vi "Main.vi"(11 "Module Admin":refnum<class "Delacor_lib_QMH_Cloneable Module Admin.lvclass">) -> ()   [LabVIEW 2019, in "moduloDqmh.lvlib"]
doc: "This template is based off of the Queued Message Handler design pattern and the Queued Message Handler project template that ships with LabVIEW.\n\nThe main difference is that the queue is private to this module and communication between modules is performed via Broadcast and Request events.\n\nRequest events are wrapped in public API methods and are handled in the Event Handling Loop (EHL) of this VI. Any module can register for Broadcast events sent by this module. The EHL generates messages based on user interface actions.\n\nThe Message Handling Loop (MHL) processes messages generated by the EHL, or by other messages. The messages are string values, so new messages can be added easily to the Message Cases case structure in the MHL. Each message cluster can also provide an optional value for Message Data, which is a variant that can be converted to whatever message-specific data is required.\n_____\nBased on Delacor QMH Project Template 5.0.0.82."
uses:
  moduloDqmh.lvlib
  <vilib>/Delacor/Delacor QMH/Libraries/Cloneable Module Admin_class/Delacor_lib_QMH_Cloneable Module Admin.lvclass
  C:/Program Files (x86)/National Instruments/LabVIEW 2019/vi.lib/Delacor/Delacor QMH/Libraries/Module Admin_class/Delacor_lib_QMH_Module Admin.lvclass
  Control 14.ctl
  Module Data--cluster.ctl
  <vilib>/Delacor/Delacor QMH/Libraries/Cloneable Module Admin_class/Delacor_lib_QMH_Cloneable Module Admin.lvclass/Delacor_lib_QMH_Cloneable Module Admin.ctl
  READ ADC Argument--cluster.ctl
  <vilib>/Delacor/Delacor QMH/Libraries/Message Queue_class/Delacor_lib_QMH_Message Queue.lvclass/Delacor_lib_QMH_Message Queue.ctl
  Read Port Argument--cluster.ctl
  Read Pin Argument--cluster.ctl
  Write Port Argument--cluster.ctl
  Write Pin Argument--cluster.ctl
  Stop Argument--cluster.ctl
  <vilib>/Delacor/Delacor QMH/Libraries/Module Admin_class/Delacor_lib_QMH_Module Admin.lvclass/Delacor_lib_QMH_Module Admin.ctl
  Arduino.lvclass
  E:/7to semestre/instrumentacion virtual/proyecto final/proyecto-final/Serial Device.lvclass
  NXP.lvclass
  simulado.lvclass
  <vilib>/Delacor/Delacor QMH/Libraries/Cloneable Module Admin_class/Delacor_lib_QMH_Get Module ID.vi
  <vilib>/Delacor/Delacor QMH/Libraries/Message Queue_class/Delacor_lib_QMH_Enqueue Message (Single).vi
  <vilib>/Delacor/Delacor QMH/Libraries/Module Admin_class/Delacor_lib_QMH_Get External Launch.vi
  <vilib>/Utility/error.llb/Error Cluster From Error Code.vi
  <vilib>/ErrorRing/Error Ring.xnode
  <vilib>/Delacor/Delacor QMH/Libraries/Message Queue_class/Delacor_lib_QMH_Message Queue.lvclass
  Serial Device.lvclass
panel:
  in  "VISA COM PORT":refnum<visa-resource-name>
  in  "Serial device Brand":T1
  in  "Config":bool
  out "Respuesta":string
  in  "CANAL":dbl
  in  "READ ADC":bool
  in  "VALOR":string
  in  "PORT":dbl
  in  "SET PORT":bool
  out "Array":bool[](array[boolean])
  in  "PORT 2":dbl
  in  "READ PORT":bool
  in  "Value":bool
  in  "PIN":dbl
  in  "PORT":dbl
  in  "SET PIN":bool
  out "Status":string
  out "Value PIN":bool
  in  "PIN":dbl
  in  "PORT":dbl
  in  "READ PIN":bool
  out "error out":errorcluster
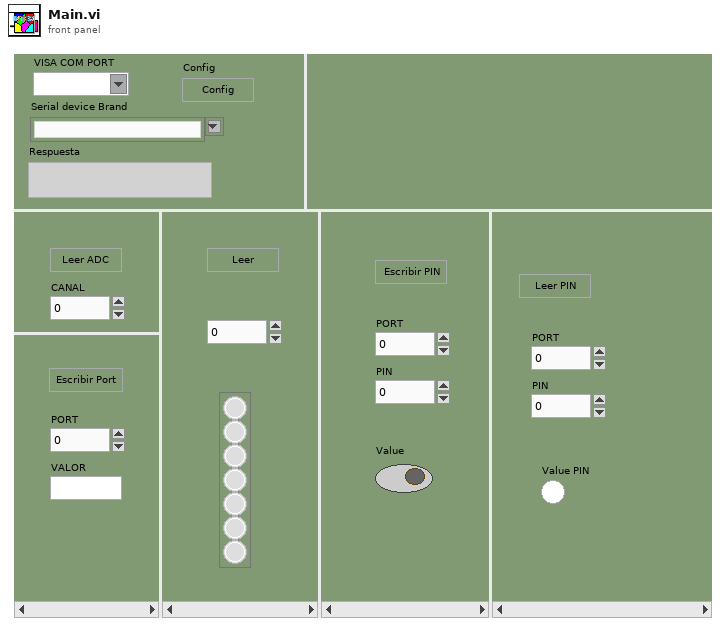
[diagram p1: front panel]
types:
  T1 = typedef "Serial Device.lvclass/Control 14.ctl" = string
  T2 = typedef "moduloDqmh.lvlib/Request Events--cluster.ctl" = cluster{"Stop Module":refnum<user-event>, "Show Panel":refnum<user-event>, "Hide Panel":refnum<user-event>, "Show Diagram":refnum<user-event>, "Get Module Execution Status":refnum<user-event>, "READ ADC":refnum<user-event>, "Read Port":refnum<user-event>, "Read Pin":refnum<user-event>, "Write Port":refnum<user-event>, "Write Pin":refnum<user-event>}
  T3 = typedef "moduloDqmh.lvlib/Module Data--cluster.ctl" = cluster{"Status":string}
  T4 = typedef "moduloDqmh.lvlib/READ ADC Argument--cluster.ctl" = cluster{"Module ID":i32, "CANAL":dbl}
  T5 = typedef "moduloDqmh.lvlib/Read Port Argument--cluster.ctl" = cluster{"Module ID":i32, "PORT 2":dbl}
  T6 = typedef "moduloDqmh.lvlib/Read Pin Argument--cluster.ctl" = cluster{"Module ID":i32, "PIN 2":dbl, "Port 4":dbl}
  T7 = typedef "moduloDqmh.lvlib/Write Port Argument--cluster.ctl" = cluster{"Module ID":i32, "String":string, "Numeric":dbl}
  T8 = typedef "moduloDqmh.lvlib/Write Pin Argument--cluster.ctl" = cluster{"Module ID":i32, "Port 3":dbl, "Pin":dbl, "Value":bool}
  T9 = enum32{"invalid lock state", "Not Locked", "Locked (No Password)", "Password-protected"}
  T10 = typedef "moduloDqmh.lvlib/Stop Argument--cluster.ctl" = cluster{"Module ID":i32, "Origin":string, "Exit via Stop Module Req?":bool, "Wait for Module to stop?":bool}
  T11 = enum32{"Invalid", "Standard", "Closed", "Hidden", "Minimized", "Maximized"}
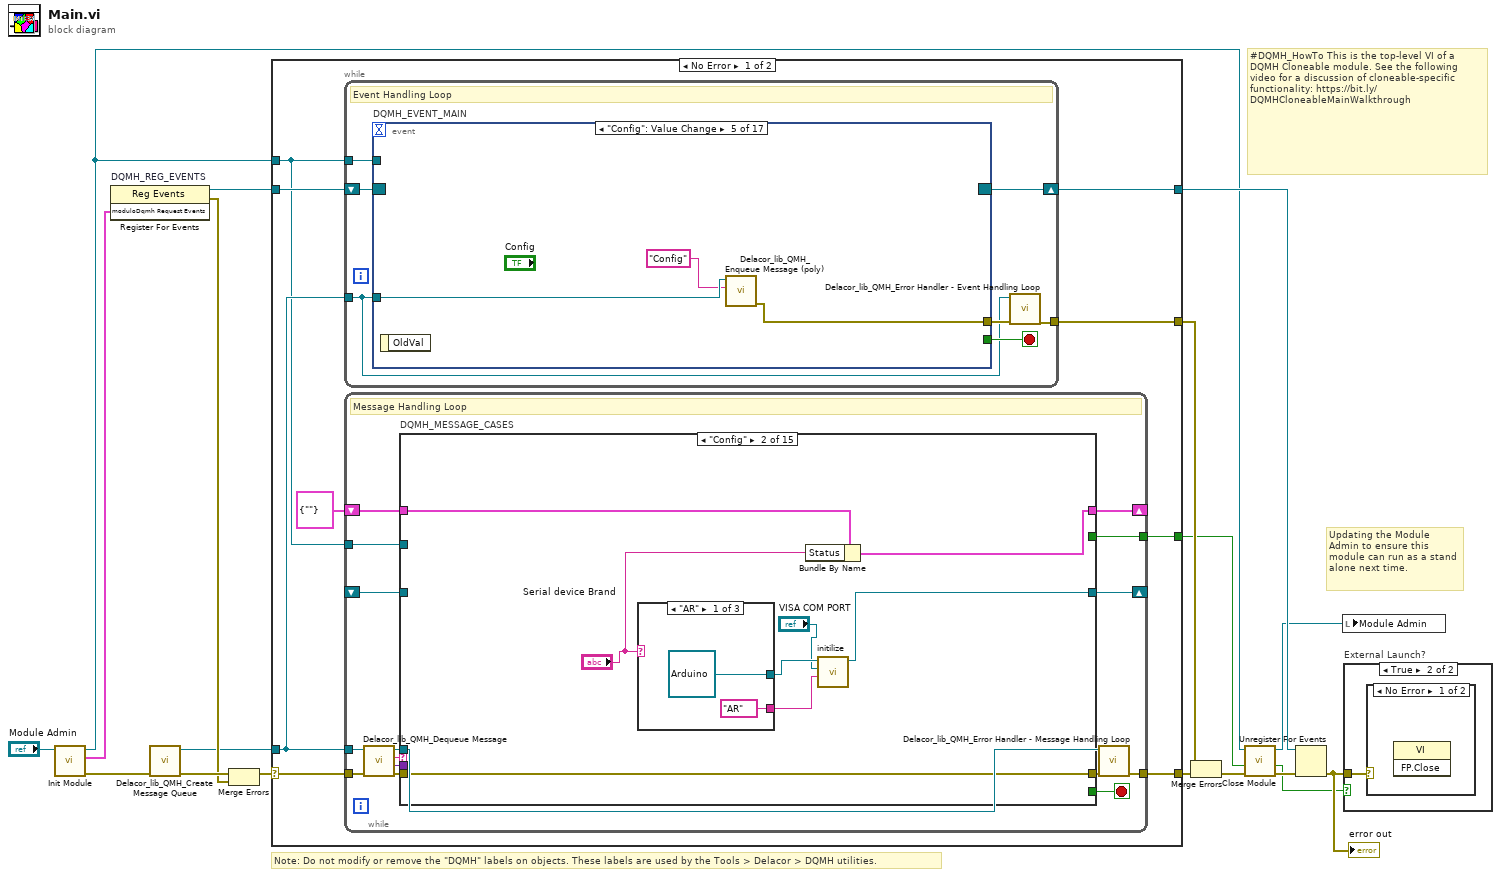
[diagram p0: block diagram]
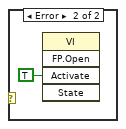
[diagram p3: hidden frame]
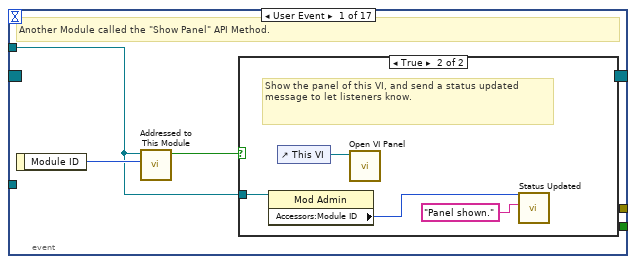
[diagram p4: hidden frame]
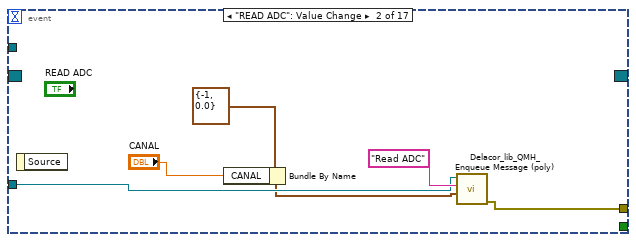
[diagram p6: hidden frame]
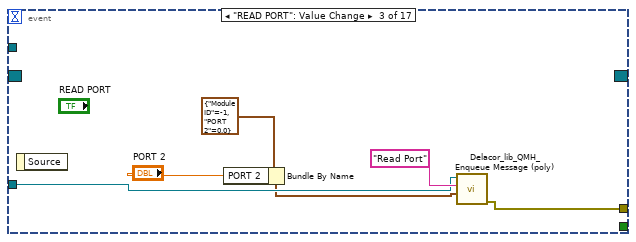
[diagram p7: hidden frame]
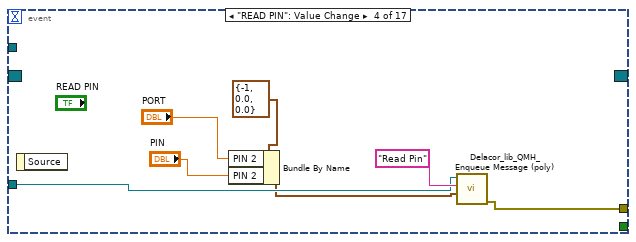
[diagram p8: hidden frame]
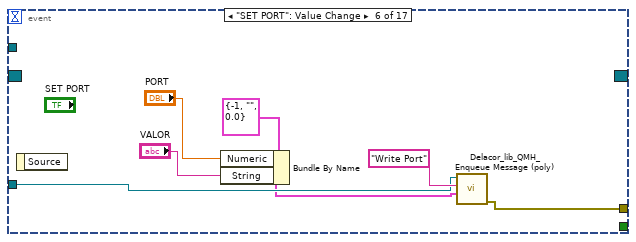
[diagram p9: hidden frame]
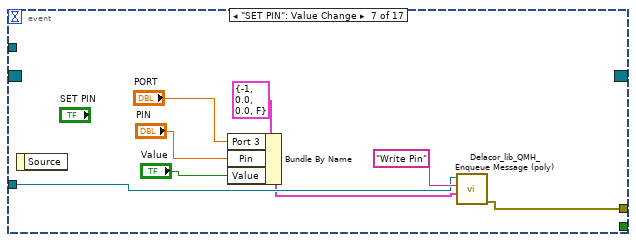
[diagram p10: hidden frame]
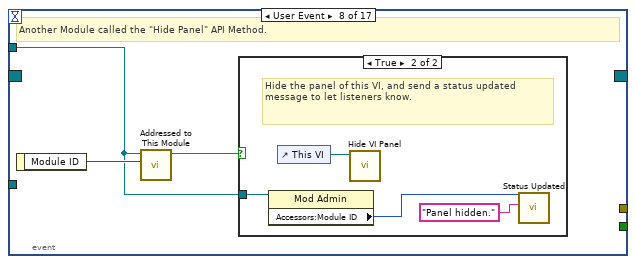
[diagram p11: hidden frame]
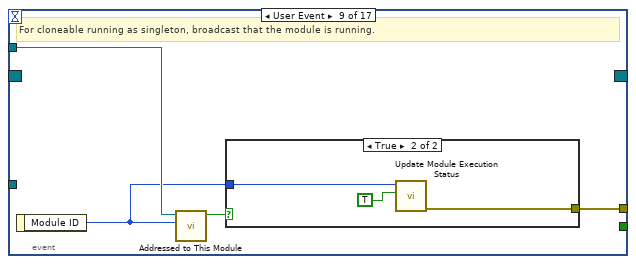
[diagram p13: hidden frame]
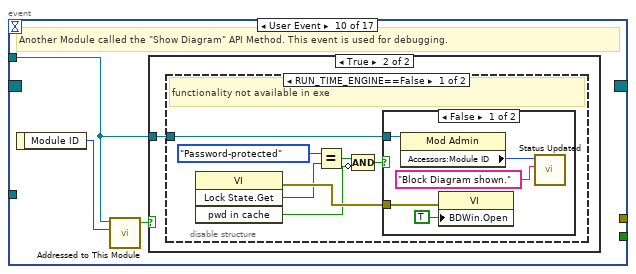
[diagram p15: hidden frame]
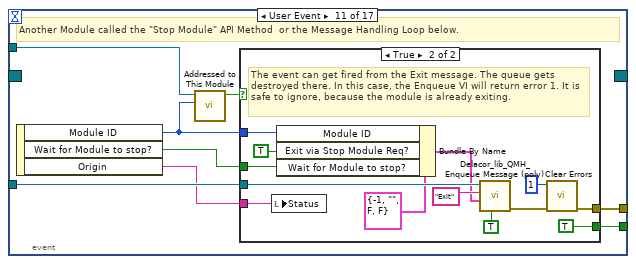
[diagram p19: hidden frame]
diagram:
  # "#DQMH_HowTo This is the top-level VI of a DQMH Cloneable module. See the following video for a discussion of cloneable-specific functionality: https://bit.ly/DQMHCloneableMainWalkthrough"
  # "Note: Do not modify or remove the \"DQMH\" labels on objects. These labels are used by the Tools > Delacor > DQMH utilities."
  # "Updating the Module Admin to ensure this module can run as a stand alone next time."
  n1 = call "Init Module.vi"("Cloneable Module Admin in"="Module Admin") -> ("error out"=w15:errorcluster, "moduloDqmh Request Events"=w7:T2, "Cloneable Module Admin out"=w4:refnum<class "Delacor_lib_QMH_Cloneable Module Admin.lvclass">)  [unwired: 8 in]
  n2 = register-events "DQMH_REG_EVENTS"(w7) -> (reference out=w8:refnum<event-registration>, error out=w10:errorcluster)  [unwired: 2 in]
  n3 = call <vilib>:"Delacor_lib_QMH_Create Message Queue.vi"("error in (no error)"=w15) -> ("error out"=w12:errorcluster, "Message Queue"=w6:refnum<class "Delacor_lib_QMH_Message Queue.lvclass">)  [unwired: 9 in]
  n4 = Merge Errors(w12, w10) -> (w11:errorcluster)
  n5 = case shown="No Error" w11 {
    selector: w11 -> [w25 w429]
    tunnel: [w27 w428] -> w16
    tunnel: [w24 w436] -> w9
    tunnel: w8 -> [w22 w436]
    tunnel: w6 -> [w21 w427]
    tunnel: [w26 _] -> w17
    tunnel: w4 -> [w20 w432]
    tunnel: [w19 _] -> w2
    frame No Error {
      n6 = while {
        tunnel: w21 -> [w28]
        shift-right: [w31] -> w24
        shift-left: w22 -> [w32]
        tunnel: [w33] -> w26
        tunnel: w20 -> [w29]
        stop <- w30 stop-if-true
        # "Event Handling Loop"
        n7 = event "DQMH_EVENT_MAIN" shown="[4] \"Config\": Value Change" {
          selector: w32 -> [_ _ _ _ _ _ _ _ _ _ _ _ _ _ _ _ _]
          dyn-events: [_ _ _ _ _ _ _ _ _ _ _ _ _ _ _ _ _] -> w31
          timeout: _ -> [_ _ _ _ _ _ _ _ _ _ _ _ _ _ _ _ _]
          tunnel: [_ _ _ _ _ _ _ _ _ _ w112 _ _ _ _ _ _] -> w30
          tunnel: w28 -> [_ w46 w52 w59 w62 w69 w77 _ _ _ w115 w131 w147 w159 w172 w185 w199]
          tunnel: [_ w45 w51 w58 w63 w68 w76 _ w89 _ w116 w134 w140 w152 w164 w177 w190] -> w34
          tunnel: w29 -> [w35 _ _ _ _ _ _ w79 w87 w93 w114 w132 w145 w157 w170 w183 w197]
          event User Event {
            # "Another Module called the \"Show Panel\" API Method."
            n8 = event-data() -> ("Module ID"=w36:i32)  [unwired: 1 in]
            n9 = call "Addressed to This Module.vi"("Module ID from Argument"=w36, "Module Admin"=w35) -> ("Addressed to this instance?"=w37:bool)  [unwired: 8 in, 1 out]
            n10 = case shown="True" w37 {
              tunnel: w35 -> [_ w39]
              frame False {
              }
              frame True {
                # "Show the panel of this VI, and send a status updated message to let listeners know."
                n11 = property class="Mod Admin"(reference=w39) -> ("Accessors:Module ID"=w38:i32)  [unwired: 1 in, 2 out]
                n12 = control-ref of="This VI"() -> (w41:refnum<vi>)
                n13 = call "Open VI Panel.vi"("VI"=w41) -> ()  [unwired: 10 in, 1 out]
                n14 = call "Status Updated.vi"("Status"="Panel shown." ("format string"), "Module ID"=w38) -> ()  [unwired: 9 in, 1 out]
              }
            }
          }
          event "READ ADC": Value Change {
            n15 = event-data() -> ()  [unwired: 1 in, 1 out]
            n16 = Bundle By Name(cluster=T4 {"Module ID"=-1, "CANAL"=0.0} ("READ ADC Argument"), "CANAL"="CANAL") -> (w43:T4)
            n17 = call-poly <vilib>:"Delacor_lib_QMH_Enqueue Message (poly).vi"("Message Data"=w43, "Message"="Read ADC", "Message Queue in"=w46) -> ("error out"=w45:errorcluster)  [unwired: 7 in, 1 out]
          }
          event "READ PORT": Value Change {
            n18 = event-data() -> ()  [unwired: 1 in, 1 out]
            n19 = Bundle By Name(cluster=T5 {"Module ID"=-1, "PORT 2"=0.0} ("Read Port Argument"), "PORT 2"="PORT 2") -> (w50:T5)
            n20 = call-poly <vilib>:"Delacor_lib_QMH_Enqueue Message (poly).vi"("Message Data"=w50, "Message"="Read Port", "Message Queue in"=w52) -> ("error out"=w51:errorcluster)  [unwired: 7 in, 1 out]
          }
          event "READ PIN": Value Change {
            n21 = event-data() -> ()  [unwired: 1 in, 1 out]
            n22 = Bundle By Name(cluster=T6 {"Module ID"=-1, "PIN 2"=0.0, "Port 4"=0.0} ("Read Pin Argument"), "PIN 2"="PORT", "PIN 2"="PIN") -> (w57:T6)
            n23 = call-poly <vilib>:"Delacor_lib_QMH_Enqueue Message (poly).vi"("Message Data"=w57, "Message"="Read Pin", "Message Queue in"=w59) -> ("error out"=w58:errorcluster)  [unwired: 7 in, 1 out]
          }
          event "Config": Value Change {
            n24 = event-data() -> ()  [unwired: 1 in, 1 out]
            n25 = call-poly <vilib>:"Delacor_lib_QMH_Enqueue Message (poly).vi"("Message"="Config", "Message Queue in"=w62) -> ("error out"=w63:errorcluster)  [unwired: 8 in, 1 out]
          }
          event "SET PORT": Value Change {
            n26 = event-data() -> ()  [unwired: 1 in, 1 out]
            n27 = Bundle By Name(cluster=T7 {"Module ID"=-1, "String"="", "Numeric"=0.0} ("Write Port Argument"), "Numeric"="PORT", "String"="VALOR") -> (w67:T7)
            n28 = call-poly <vilib>:"Delacor_lib_QMH_Enqueue Message (poly).vi"("Message Data"=w67, "Message"="Write Port", "Message Queue in"=w69) -> ("error out"=w68:errorcluster)  [unwired: 7 in, 1 out]
          }
          event "SET PIN": Value Change {
            n29 = event-data() -> ()  [unwired: 1 in, 1 out]
            n30 = Bundle By Name(cluster=T8 {"Module ID"=-1, "Port 3"=0.0, "Pin"=0.0, "Value"=FALSE} ("Write Pin Argument"), "Port 3"="PORT", "Pin"="PIN", "Value"="Value") -> (w75:T8)
            n31 = call-poly <vilib>:"Delacor_lib_QMH_Enqueue Message (poly).vi"("Message Data"=w75, "Message"="Write Pin", "Message Queue in"=w77) -> ("error out"=w76:errorcluster)  [unwired: 7 in, 1 out]
          }
          event User Event {
            # "Another Module called the \"Hide Panel\" API Method."
            n32 = event-data() -> ("Module ID"=w80:i32)  [unwired: 1 in]
            n33 = call "Addressed to This Module.vi"("Module ID from Argument"=w80, "Module Admin"=w79) -> ("Addressed to this instance?"=w81:bool)  [unwired: 8 in, 1 out]
            n34 = case shown="True" w81 {
              tunnel: w79 -> [_ w83]
              frame False {
              }
              frame True {
                # "Hide the panel of this VI, and send a status updated message to let listeners know."
                n35 = property class="Mod Admin"(reference=w83) -> ("Accessors:Module ID"=w82:i32)  [unwired: 1 in, 2 out]
                n36 = control-ref of="This VI"() -> (w85:refnum<vi>)
                n37 = call "Hide VI Panel.vi"("VI"=w85) -> ()  [unwired: 10 in, 1 out]
                n38 = call "Status Updated.vi"("Status"="Panel hidden." ("format string"), "Module ID"=w82) -> ()  [unwired: 9 in, 1 out]
              }
            }
          }
          event User Event {
            # "For cloneable running as singleton, broadcast that the module is running."
            n39 = event-data() -> ("Module ID"=w86:i32)  [unwired: 1 in]
            n40 = call "Addressed to This Module.vi"("Module ID from Argument"=w86, "Module Admin"=w87) -> ("Addressed to this instance?"=w88:bool)  [unwired: 8 in, 1 out]
            n41 = case shown="True" w88 {
              tunnel: [_ w92] -> w89
              tunnel: w86 -> [_ w91]
              frame False {
              }
              frame True {
                n42 = call "Update Module Execution Status.vi"("Running?"=TRUE, "Module ID"=w91) -> ("error out"=w92:errorcluster)  [unwired: 9 in]
              }
            }
          }
          event User Event {
            # "Another Module called the \"Show Diagram\" API Method. This event is used for debugging."
            n43 = event-data() -> ("Module ID"=w94:i32)  [unwired: 1 in]
            n44 = call "Addressed to This Module.vi"("Module ID from Argument"=w94, "Module Admin"=w93) -> ("Addressed to this instance?"=w95:bool)  [unwired: 8 in, 1 out]
            n45 = case shown="True" w95 {
              tunnel: w93 -> [_ w96]
              frame False {
              }
              frame True {
                n46 = disable-structure shown="RUN_TIME_ENGINE==False" {
                  disable-tunnel: w96 -> [w97 _]
                  frame condition #0 (active) {
                    # "functionality not available in exe"
                    n47 = invoke class="VI" method="Lock State.Get"() -> (error out=w103:errorcluster, "Get Lock State"=w102:T9, "pwd in cache"=w99:bool)  [unwired: 4 in, 1 out]
                    n48 = Equal?(x=T9."Password-protected", y=w102) -> (x = y?=w100:bool)
                    n49 = Compound Arithmetic op=AND(w100, invert w99) -> (w98:bool)
                    n50 = case shown="False" w98 {
                      tunnel: w103 -> [w108 _]
                      tunnel: w97 -> [w105 _]
                      frame False {
                        n51 = property class="Mod Admin"(reference=w105) -> ("Accessors:Module ID"=w104:i32)  [unwired: 1 in, 2 out]
                        n52 = property class="VI"(error in=w108, "BDWin.Open"=TRUE ("Block Diagram Window:Open")) -> ()  [unwired: 1 in, 2 out]
                        n53 = call "Status Updated.vi"("Status"="Block Diagram shown." ("format string"), "Module ID"=w104) -> ()  [unwired: 9 in, 1 out]
                      }
                      frame True {
                        # "Password-protected VI, and the password is not in the cache. Do not show the diagram."
                      }
                    }
                  }
                  frame condition #1 {
                  }
                }
              }
            }
          }
          event User Event {
            # "Another Module called the \"Stop Module\" API Method  or the Message Handling Loop below."
            n54 = event-data() -> ("Module ID"=w110:i32, "Wait for Module to stop?"=w111:bool, "Origin"=w109:string)  [unwired: 1 in]
            n55 = call "Addressed to This Module.vi"("Module ID from Argument"=w110, "Module Admin"=w114) -> ("Addressed to this instance?"=w113:bool)  [unwired: 8 in, 1 out]
            n56 = case shown="True" w113 {
              tunnel: [_ w128] -> w116
              tunnel: w115 -> [_ w124]
              tunnel: [_ TRUE] -> w112
              tunnel: w111 -> [_ w119]
              tunnel: w110 -> [_ w121]
              tunnel: w109 -> [_ w117]
              frame False {
              }
              frame True {
                # "The event can get fired from the Exit message. The queue gets destroyed there. In this case, the Enqueue VI will return error 1. It is safe to ignore, because the module is already exiting."
                n57 = local write "Status"(w117) -> ()
                n58 = Bundle By Name(cluster=T10 {"Module ID"=-1, "Origin"="", "Exit via Stop Module Req?"=FALSE, "Wait for Module to stop?"=FALSE} ("Stop Argument"), "Module ID"=w121, "Exit via Stop Module Req?"=TRUE, "Wait for Module to stop?"=w119) -> (w118:T10)
                n59 = call-poly <vilib>:"Delacor_lib_QMH_Enqueue Message (poly).vi"("Priority Message? (F)"=TRUE, "Message Data"=w118, "Message"="Exit", "Message Queue in"=w124) -> ("error out"=w129:errorcluster)  [unwired: 6 in, 1 out]
                n60 = call <vilib>:"Clear Errors.vi"("error in (no error)"=w129, "specific error code to clear (0: all)"=1) -> ("error out"=w128:errorcluster)  [unwired: 4 in, 1 out]
              }
            }
          }
          event Panel Close? {
            w133 = TRUE  # Discard the event, the MHL is responsible for closing and stopping this VI.
            # "Hide the panel or send the 'Exit' message if the user clicks the 'X' on the module main VI panel."
            n61 = event-data() -> ()  [unwired: 1 in, 1 out]
            n62 = property class="Mod Admin"(reference=w132) -> ("Accessors:External Launch"=w130:bool)  [unwired: 1 in, 2 out]
            n63 = case shown="False" w130 {
              tunnel: w131 -> [_ w138]
              tunnel: [_ w139] -> w134
              frame True {
                # "If externally launched, clicking the 'X' hides the panel, but doesn't close it."
                n64 = control-ref of="This VI"() -> (w135:refnum<vi>)
                n65 = call "Hide VI Panel.vi"("VI"=w135) -> ()  [unwired: 10 in, 1 out]
              }
              frame False {
                # "If run as a stand-alone VI, clicking the panel 'X' stops the VI."
                n66 = call-poly <vilib>:"Delacor_lib_QMH_Enqueue Message (poly).vi"("Priority Message? (F)"=TRUE, "Message"="Exit", "Message Queue in"=w138) -> ("error out"=w139:errorcluster)  [unwired: 7 in, 1 out]
              }
            }
            n67 = event-data("Discard?"=w133) -> ()  [unwired: 1 in, 1 out]
          }
          event User Event {
            # "Another Module called the \"READ ADC\" API Method."
            n68 = event-data() -> ("Module ID"=w142:i32, "CANAL"=w141:dbl)  [unwired: 1 in]
            n69 = Bundle(cluster=T4 {"Module ID"=-1, "CANAL"=0.0} ("READ ADC Argument"), "Module ID"=w142, "CANAL"=w141) -> (w143:T4)
            n70 = call "Addressed to This Module.vi"("Module ID from Argument"=w142, "Module Admin"=w145) -> ("Addressed to this instance?"=w146:bool)  [unwired: 8 in, 1 out]
            n71 = case shown="True" w146 {
              tunnel: w147 -> [_ w151]
              tunnel: w143 -> [_ w149]
              tunnel: [_ w148] -> w140
              frame False {
              }
              frame True {
                n72 = call-poly <vilib>:"Delacor_lib_QMH_Enqueue Message (poly).vi"("Message Data"=w149, "Message"="READ ADC", "Message Queue in"=w151) -> ("error out"=w148:errorcluster)  [unwired: 7 in, 1 out]
              }
            }
          }
          event User Event {
            # "Another Module called the \"Read Port\" API Method."
            n73 = event-data() -> ("Module ID"=w154:i32, "PORT 2"=w153:dbl)  [unwired: 1 in]
            n74 = Bundle(cluster=T5 {"Module ID"=-1, "PORT 2"=0.0} ("Read Port Argument"), "Module ID"=w154, "PORT 2"=w153) -> (w155:T5)
            n75 = call "Addressed to This Module.vi"("Module ID from Argument"=w154, "Module Admin"=w157) -> ("Addressed to this instance?"=w158:bool)  [unwired: 8 in, 1 out]
            n76 = case shown="True" w158 {
              tunnel: w159 -> [_ w163]
              tunnel: w155 -> [_ w161]
              tunnel: [_ w160] -> w152
              frame False {
              }
              frame True {
                n77 = call-poly <vilib>:"Delacor_lib_QMH_Enqueue Message (poly).vi"("Message Data"=w161, "Message"="Read Port", "Message Queue in"=w163) -> ("error out"=w160:errorcluster)  [unwired: 7 in, 1 out]
              }
            }
          }
          event User Event {
            # "Another Module called the \"Read Pin\" API Method."
            n78 = event-data() -> ("Module ID"=w167:i32, "PIN 2"=w166:dbl, "Port 4"=w165:dbl)  [unwired: 1 in]
            n79 = Bundle(cluster=T6 {"Module ID"=-1, "PIN 2"=0.0, "Port 4"=0.0} ("Read Pin Argument"), "Module ID"=w167, "PIN 2"=w166, "Port 4"=w165) -> (w168:T6)
            n80 = call "Addressed to This Module.vi"("Module ID from Argument"=w167, "Module Admin"=w170) -> ("Addressed to this instance?"=w171:bool)  [unwired: 8 in, 1 out]
            n81 = case shown="True" w171 {
              tunnel: w172 -> [_ w176]
              tunnel: w168 -> [_ w174]
              tunnel: [_ w173] -> w164
              frame False {
              }
              frame True {
                n82 = call-poly <vilib>:"Delacor_lib_QMH_Enqueue Message (poly).vi"("Message Data"=w174, "Message"="Read Pin", "Message Queue in"=w176) -> ("error out"=w173:errorcluster)  [unwired: 7 in, 1 out]
              }
            }
          }
          event User Event {
            # "Another Module called the \"Write Port\" API Method."
            n83 = event-data() -> ("Module ID"=w180:i32, "String"=w179:string, "Numeric"=w178:dbl)  [unwired: 1 in]
            n84 = Bundle(cluster=T7 {"Module ID"=-1, "String"="", "Numeric"=0.0} ("Write Port Argument"), "Module ID"=w180, "String"=w179, "Numeric"=w178) -> (w181:T7)
            n85 = call "Addressed to This Module.vi"("Module ID from Argument"=w180, "Module Admin"=w183) -> ("Addressed to this instance?"=w184:bool)  [unwired: 8 in, 1 out]
            n86 = case shown="True" w184 {
              tunnel: w185 -> [_ w189]
              tunnel: w181 -> [_ w187]
              tunnel: [_ w186] -> w177
              frame False {
              }
              frame True {
                n87 = call-poly <vilib>:"Delacor_lib_QMH_Enqueue Message (poly).vi"("Message Data"=w187, "Message"="Write Port", "Message Queue in"=w189) -> ("error out"=w186:errorcluster)  [unwired: 7 in, 1 out]
              }
            }
          }
          event User Event {
            # "Another Module called the \"Write Pin\" API Method."
            n88 = event-data() -> ("Module ID"=w194:i32, "Port 3"=w193:dbl, "Pin"=w192:dbl, "Value"=w191:bool)  [unwired: 1 in]
            n89 = Bundle(cluster=T8 {"Module ID"=-1, "Port 3"=0.0, "Pin"=0.0, "Value"=FALSE} ("Write Pin Argument"), "Module ID"=w194, "Port 3"=w193, "Pin"=w192, "Value"=w191) -> (w195:T8)
            n90 = call "Addressed to This Module.vi"("Module ID from Argument"=w194, "Module Admin"=w197) -> ("Addressed to this instance?"=w198:bool)  [unwired: 8 in, 1 out]
            n91 = case shown="True" w198 {
              tunnel: w199 -> [_ w203]
              tunnel: w195 -> [_ w201]
              tunnel: [_ w200] -> w190
              frame False {
              }
              frame True {
                n92 = call-poly <vilib>:"Delacor_lib_QMH_Enqueue Message (poly).vi"("Message Data"=w201, "Message"="Write Pin", "Message Queue in"=w203) -> ("error out"=w200:errorcluster)  [unwired: 7 in, 1 out]
              }
            }
          }
        }
        n93 = call-dynamic "Delacor_lib_QMH_Error Handler - Event Handling Loop.vi"("error in (no error)"=w34, "Message Queue in"=w28) -> ("dup error in"=w33:errorcluster)  [unwired: 8 in, 1 out]
      }
      n94 = while {
        tunnel: w21 -> [w209]
        shift-right: [w213] -> _
        shift-left: T3 {"Status"=""} ("Data Cluster") -> [w214]
        tunnel: w25 -> [w217]
        tunnel: [w215] -> w27
        tunnel: w20 -> [w207]
        tunnel: [w206] -> w19
        shift-right: [w205] -> _
        shift-left: _ -> [w204]
        stop <- w212 stop-if-true
        # "Message Handling Loop"
        n95 = call-dynamic "Delacor_lib_QMH_Dequeue Message.vi"("error in (no error)"=w217, "Message Queue in"=w209) -> ("error out"=w216:errorcluster, "Message Data"=w210:variant, "Message"=w211:string, "Message Queue out"=w208:refnum<class "Delacor_lib_QMH_Message Queue.lvclass">)  [unwired: 6 in]
        n96 = case "DQMH_MESSAGE_CASES" shown="\"Config\"" w211 {
          selector: w211 -> [_ _ _ _ _ _ _ _ _ _ _ _ _ _ w414]
          tunnel: w208 -> [_ _ _ _ w266 _ w300 w320 w336 _ _ w362 _ w403 _]
          tunnel: w216 -> [w235 w245 w254 w262 w279 w295 w316 w333 w351 w355 w358 w371 w385 w409 w416]
          tunnel: [w233 w245 w254 w257 w268 w284 w303 w317 w338 w354 w358 w367 w384 w406 w417] -> w218
          tunnel: w214 -> [w226 w240 w253 w261 w278 w294 w315 w332 w350 w353 w357 w366 w382 w402 w415]
          tunnel: [w226 w239 w253 w261 w278 w294 w315 w332 w350 w353 w357 w366 w382 w402 w415] -> w213
          tunnel: [_ _ _ _ _ _ _ _ _ _ _ _ _ w401 _] -> w212
          tunnel: w210 -> [_ _ _ w260 w277 w293 w314 w331 w349 _ _ w365 _ w399 _]
          tunnel: w207 -> [w221 _ _ _ _ _ _ _ _ _ _ w364 w380 w395 w412]
          tunnel: [_ _ _ _ _ _ _ _ _ _ _ _ _ w397 _] -> w206
          tunnel: [w219 w241 w252 w259 w272 w288 w309 w323 w344 w352 w356 w359 w378 w393 w410] -> w205
          tunnel: w204 -> [w219 _ w252 w259 w274 w290 w311 w327 w346 w352 w356 w359 w378 w393 w410]
          frame "Initialize" {
            # "Initialize - Any operation that needs to be done before the module can receive messages. Synchronize Caller Events.vi will inform Start Module.vi that the module has launched and is ready to receive messages. Module Did Init.vi will broadcast that the module initialized."
            n97 = call "Synchronize Caller Events.vi"("error in (no error)"=w235, "Module Admin"=w221) -> ("error out"=w234:errorcluster, "Module Admin out"=w220:refnum<class "Delacor_lib_QMH_Cloneable Module Admin.lvclass">)  [unwired: 8 in]
            n98 = property class="Mod Admin"(reference=w220) -> ("Accessors:Module ID"=w223:i32, "Accessors:External Launch"=w222:bool)  [unwired: 1 in, 2 out]
            n99 = call "Module Name--constant.vi"("Module ID"=w223) -> ("Module Name"=w230:string)  [unwired: 10 in]
            n100 = property class="VI"("Front Panel.Title"=w230) -> (reference out=w232:refnum<vi>, error out=w237:errorcluster)  [unwired: 2 in]
            n101 = Select(t=T11."Hidden" ("State"), s=w222, f=T11."Standard" ("State")) -> (s? t:f=w227:T11)
            n102 = invoke class="VI" method="FP.Open"(reference=w232, error in=w237, "State"=w227) -> (reference out=w231:refnum<vi>, error out=w236:errorcluster)  [unwired: 2 in, 3 out]
            n103 = call "Module Name--constant.vi"("Module ID"=w223) -> ("Module Name"=w224:string)  [unwired: 10 in]
            n104 = invoke class="VI" method="FP.Center"(reference=w231, error in=w236) -> ()  [unwired: 1 in, 3 out]
            n105 = call "Module Did Init.vi"("error in (no error)"=w234, "Initialized?"=TRUE, "Origin"=w224, "Module ID"=w223) -> ("error out"=w233:errorcluster)  [unwired: 7 in]
          }
          frame "Config" {
            n106 = case shown="\"AR\"" "Serial device Brand" {
              tunnel: [refnum<class "Arduino.lvclass"> refnum ("Arduino.lvclass") refnum<class "NXP.lvclass"> refnum ("NXP.lvclass") w251] -> w243
              tunnel: [T1 "AR" ("Serial device Brand") T1 "NX" ("Serial device Brand") T1 "SD" ("Serial device Brand")] -> w244
              frame "AR" {
              }
              frame "NX" {
              }
              frame "SD", Default {
                w251 = refnum<class "simulado.lvclass"> refnum  # simulado.lvclass
              }
            }
            n107 = Bundle By Name(cluster=w240, "Status"="Serial device Brand") -> (w239:T3)
            n108 = call-dynamic "initilize.vi"("Serial device Brand"=w244, "VISA resource name"="VISA COM PORT", "Serial Device in"=w243) -> ("Serial Device out"=w241:refnum<class "Serial Device.lvclass">)  [unwired: 7 in, 1 out]
          }
          frame "--- Module Specific ---" {
            # "Separator -- The following cases handle messages specific to this Module."
          }
          frame "Respuesta" {
            # "LECTURA ADC"
            n109 = Variant To Data(error in=w262, type="", Variant=w260) -> (data=→"Respuesta":string, error out=w258:errorcluster)
            n110 = Merge Errors(w258) -> (w257:errorcluster)
          }
          frame "READ ADC" {
            # "LECTURA ADC"
            n111 = Variant To Data(error in=w279, type=T4 {"Module ID"=-1, "CANAL"=0.0} ("READ ADC Argument"), Variant=w277) -> (data=w275:T4, error out=w269:errorcluster)
            n112 = Unbundle By Name(w275) -> ("CANAL"=w271:dbl)  [unwired: 1 out]
            n113 = call-dynamic "Read ADC.vi"("canal"=w271, "Serial Device in"=w274) -> ("error out"=w270:errorcluster, "Serial Device out"=w273:refnum<class "Serial Device.lvclass">)  [unwired: 8 in]
            n114 = call-dynamic "respuesta read adc.vi"("error in (no error)"=w270, "Serial Device in"=w273) -> ("error out"=w267:errorcluster, "salida"=w265:string, "Serial Device out"=w272:refnum<class "Serial Device.lvclass">)  [unwired: 7 in]
            n115 = call-poly <vilib>:"Delacor_lib_QMH_Enqueue Message (poly).vi"("error in (no error)"=w267, "Message Data"=w265, "Message"="Respuesta", "Message Queue in"=w266) -> ("error out"=w263:errorcluster)  [unwired: 6 in, 1 out]
            n116 = Merge Errors(w263, w269) -> (w268:errorcluster)
          }
          frame "Read Port" {
            # "Read port"
            n117 = Variant To Data(error in=w295, type=T5 {"Module ID"=-1, "PORT 2"=0.0} ("Read Port Argument"), Variant=w293) -> (data=w291:T5, error out=w285:errorcluster)
            n118 = Unbundle By Name(w291) -> ("PORT 2"=w287:dbl)  [unwired: 1 out]
            n119 = call-dynamic "GETPORTSTATUS.vi"("Port to read"=w287, "Serial Device in"=w290) -> ("error out"=w286:errorcluster, "Serial Device out"=w289:refnum<class "Serial Device.lvclass">)  [unwired: 8 in]
            n120 = call-dynamic "reponsegetport.vi"("error in (no error)"=w286, "Serial Device in"=w289) -> ("error out"=w283:errorcluster, "String"=w282:string, "Serial Device out"=w288:refnum<class "Serial Device.lvclass">)  [unwired: 7 in]
            n121 = Merge Errors(w283, w285) -> (w284:errorcluster)
            n122 = Hexadecimal String To Number(string=w282) -> (number=w281:u32)  [unwired: 2 in, 1 out]
            n123 = Number To Boolean Array(number=w281) -> (Boolean array=→"Array":bool[])
          }
          frame "Read Pin" {
            n124 = Variant To Data(error in=w316, type=T6 {"Module ID"=-1, "PIN 2"=0.0, "Port 4"=0.0} ("Read Pin Argument"), Variant=w314) -> (data=w312:T6, error out=w304:errorcluster)
            n125 = Unbundle By Name(w312) -> ("PIN 2"=w307:dbl, "Port 4"=w308:dbl)  [unwired: 1 out]
            n126 = call-dynamic "GETPINSTATUS.vi"("pin"=w307, "Port"=w308, "Serial Device in"=w311) -> ("error out"=w306:errorcluster, "Serial Device out"=w310:refnum<class "Serial Device.lvclass">)  [unwired: 7 in]
            n127 = call-dynamic "Getpinstatusresponse.vi"("error in (no error)"=w306, "Serial Device in"=w310) -> ("error out"=w301:errorcluster, "Value"=w296:string, "Serial Device out"=w309:refnum<class "Serial Device.lvclass">)  [unwired: 7 in]
            n128 = call-poly <vilib>:"Delacor_lib_QMH_Enqueue Message (poly).vi"("error in (no error)"=w301, "Message Data"=w296, "Message"="Respuesta", "Message Queue in"=w300) -> ("error out"=w302:errorcluster)  [unwired: 6 in, 1 out]
            n129 = Merge Errors(w302, w304) -> (w303:errorcluster)
            n130 = Decimal String To Number(string=w296) -> (number=w299:i32)  [unwired: 2 in, 1 out]
            n131 = Equal To 0?(x=w299) -> (x = 0?=w298:bool)
            n132 = Not(x=w298) -> (.not. x?=→"Value PIN":bool)
          }
          frame "Write Port" {
            n133 = Variant To Data(error in=w333, type=T7 {"Module ID"=-1, "String"="", "Numeric"=0.0} ("Write Port Argument"), Variant=w331) -> (data=w329:T7, error out=w322:errorcluster)
            n134 = Unbundle By Name(w329) -> ("Numeric"=w328:dbl, "String"=w326:string)
            n135 = call-dynamic "SETPORT.vi"("error in (no error)"=w322, "Valor"=w326, "Port"=w328, "Serial Device in"=w327) -> ("error out"=w324:errorcluster, "Serial Device out"=w325:refnum<class "Serial Device.lvclass">)  [unwired: 6 in]
            n136 = call-dynamic "respuesta read adc.vi"("error in (no error)"=w324, "Serial Device in"=w325) -> ("error out"=w321:errorcluster, "salida"=w318:string, "Serial Device out"=w323:refnum<class "Serial Device.lvclass">)  [unwired: 7 in]
            n137 = call-poly <vilib>:"Delacor_lib_QMH_Enqueue Message (poly).vi"("error in (no error)"=w321, "Message Data"=w318, "Message"="Respuesta", "Message Queue in"=w320) -> ("error out"=w317:errorcluster)  [unwired: 6 in, 1 out]
          }
          frame "Write Pin" {
            n138 = Variant To Data(error in=w351, type=T8 {"Module ID"=-1, "Port 3"=0.0, "Pin"=0.0, "Value"=FALSE} ("Write Pin Argument"), Variant=w349) -> (data=w347:T8, error out=w339:errorcluster)
            n139 = Unbundle By Name(w347) -> ("Port 3"=w343:dbl, "Pin"=w342:dbl, "Value"=w341:bool)
            n140 = call-dynamic "SETPINSTATUS.vi"("Serial Device in"=w346, "PORT"=w343, "PIN"=w342, "valor"=w341) -> ("Serial Device out"=w345:refnum<class "Serial Device.lvclass">, "error out"=w340:errorcluster)  [unwired: 10 in]
            n141 = call-dynamic "respuesta read adc.vi"("error in (no error)"=w340, "Serial Device in"=w345) -> ("error out"=w337:errorcluster, "salida"=w335:string, "Serial Device out"=w344:refnum<class "Serial Device.lvclass">)  [unwired: 7 in]
            n142 = Merge Errors(w337, w339) -> (w338:errorcluster)
            n143 = call-poly <vilib>:"Delacor_lib_QMH_Enqueue Message (poly).vi"("Message Data"=w335, "Message"="Respuesta", "Message Queue in"=w336) -> ()  [unwired: 7 in, 2 out]
          }
          frame "---Copy This Frame---" {
            # "Duplicate this frame when creating new messages.  Change this comment in the duplicated frame to describe this message."
            n144 = Merge Errors(w355) -> (w354:errorcluster)
          }
          frame "--- Exit and Error Handling---" {
            # "Separator - the following cases handle errors and exit messages."
          }
          frame "Error" {
            # "#CodeRecommended - If you ever change the name of this \"Error\" message, you'll need to update the name in the Check Loop Error.vi as well."
            # "#CodeRecommended - If the module is running in standalone mode (External Launch = FALSE), this code will pop up an error dialog and call the 'Exit' message if an error occurs. Add more fine-grained error handling here."
            # "Error - Check the error message data and respond accordingly. This message is sent by the \"Error Handler\" VIs at the end of each loop in this application."
            n145 = property class="Mod Admin"(reference=w364) -> ("Accessors:External Launch"=w363:bool, "Accessors:Module ID"=w360:i32)  [unwired: 1 in, 2 out]
            n146 = Variant To Data(error in=w371, type=errorcluster {"status"=FALSE, "code"=0, "source"=""} ("error constant"), Variant=w365) -> (data=w372:errorcluster, error out=w369:errorcluster)
            n147 = call "Module Name--constant.vi"("Module ID"=w360) -> ("Module Name"=w361:string)  [unwired: 10 in]
            n148 = call "Error Reported.vi"("Additional Information"=w361, "Error"=w372, "Module ID"=w360) -> ()  [unwired: 8 in, 1 out]
            n149 = case shown="False" w363 {
              tunnel: [w377 _] -> w368
              tunnel: w362 -> [w375 _]
              tunnel: w372 -> [w376 _]
              frame False {
                # "If the module is running standalone, then pop up an error dialog and call the \"Exit\" message."
                n150 = call <vilib>:"Simple Error Handler.vi"("error in (no error)"=w376) -> ()  [unwired: 4 in, 5 out]
                n151 = call-poly <vilib>:"Delacor_lib_QMH_Enqueue Message (poly).vi"("Priority Message? (F)"=TRUE, "Message"="Exit", "Message Queue in"=w375) -> ("error out"=w377:errorcluster)  [unwired: 7 in, 1 out]
              }
              frame True {
                # "If the module was launched externally, calling the Error Reported broadcast VI is the only action performed by the \"Error\" message. The module's caller can then process the error appropriately."
              }
            }
            n152 = Merge Errors(w369, w368) -> (w367:errorcluster)
            n153 = local write "error out"(w367) -> ()
          }
          frame "Simulate MHL Error" {
            # "#DQMH_HowTo The 'Simulate MHL Error' button  illustrates how the MHL handles errors. This event is instructional in nature and can be removed."
            # "Simulate an error occurring at the MHL"
            n154 = property class="Mod Admin"(reference=w380) -> ("Accessors:Module ID"=w381:i32)  [unwired: 1 in, 2 out]
            n155 = call "Module Name--constant.vi"("Module ID"=w381) -> ("Module Name"=w379:string)  [unwired: 10 in]
            n156 = xnode "Error Ring"("parameter 0"=w379) -> ("error out"=w383:errorcluster)
            n157 = Merge Errors(w385, w383) -> (w384:errorcluster)
          }
          frame "Exit" {
            w400 = 91  # 91: not all Exit messages will have an argument
            w401 = TRUE  # Stop the VI
            # "Release the message queue reference"
            # "#CodeNeeded - Add any required cleanup code here."
            # "Exit - Exit the application."
            n158 = Variant To Data(error in=w409, type=T10 {"Module ID"=-1, "Origin"="", "Exit via Stop Module Req?"=FALSE, "Wait for Module to stop?"=FALSE} ("Stop Argument"), Variant=w399) -> (data=w396:T10, error out=w404:errorcluster)
            n159 = call <vilib>:"Clear Errors.vi"("error in (no error)"=w404, "specific error code to clear (0: all)"=w400) -> ("error out"=w408:errorcluster)  [unwired: 4 in, 1 out]
            n160 = control-ref of="This VI"() -> (w394:refnum<vi>)
            n161 = call-dynamic "Delacor_lib_QMH_Release Message Queue.vi"("error in (no error)"=w408, "Message Queue"=w403) -> ("error out"=w407:errorcluster)  [unwired: 9 in]
            n162 = call "Handle Exit.vi"("Stop Argument"=w396, "Module Admin in"=w395, "VI reference"=w394) -> ("error out"=w405:errorcluster, "Wait for Stop?"=w397:bool)  [unwired: 7 in]
            n163 = Merge Errors(w407, w405) -> (w406:errorcluster)
          }
          frame Default {
            # "'Default' case only runs if there is a message that isn't defined in any of the other cases.  Output a programming error."
            n164 = property class="Mod Admin"(reference=w412) -> ("Accessors:Module ID"=w411:i32)  [unwired: 1 in, 2 out]
            n165 = call "Module Name--constant.vi"("Module ID"=w411) -> ("Module Name"=w413:string)  [unwired: 10 in]
            n166 = xnode "Error Ring"("parameter 0"=w414, "parameter 1"=w413) -> ("error out"=w418:errorcluster)
            n167 = Merge Errors(w416, w418) -> (w417:errorcluster)
          }
        }
        n168 = call-dynamic "Delacor_lib_QMH_Error Handler - Message Handling Loop.vi"("error in (no error)"=w218, "Message Queue in"=w208) -> ("dup error in"=w215:errorcluster)  [unwired: 8 in, 1 out]
      }
    }
    frame Error {
      n169 = call "Synchronize Caller Events.vi"("Module Admin"=w432) -> ("Module Admin out"=w431:refnum<class "Delacor_lib_QMH_Cloneable Module Admin.lvclass">)  [unwired: 9 in, 1 out]
      n170 = property class="Mod Admin"(reference=w431) -> ("Accessors:Module ID"=w430:i32)  [unwired: 1 in, 2 out]
      n171 = call-dynamic "Delacor_lib_QMH_Release Message Queue.vi"("error in (no error)"=w429, "Message Queue"=w427) -> ("error out"=w428:errorcluster)  [unwired: 9 in]
      n172 = call "Module Name--constant.vi"("Module ID"=w430) -> ("Module Name"=w435:string)  [unwired: 10 in]
      n173 = Format Into String(format string="An error occurred during initialization. %s is no longer running.", w435) -> (resulting string=w433:string)  [unwired: 2 in, 1 out]
      n174 = call "Error Reported.vi"("Additional Information"=w433, "Error"=w428, "Module ID"=w430) -> ()  [unwired: 8 in, 1 out]
    }
  }
  n175 = Merge Errors(w17, w16) -> (w18:errorcluster)
  n176 = call "Close Module.vi"("error in"=w18, "Wait for stop?"=w2, "Module Admin in"=w4) -> ("error out"=w14:errorcluster, "External Launch"=w1:bool, "Module Admin out"=w3:refnum<class "Delacor_lib_QMH_Cloneable Module Admin.lvclass">)  [unwired: 6 in]
  n177 = Unregister For Events(event registration refnum=w9, error in=w14) -> (error out=w13:errorcluster)
  "error out" <- w13
  n178 = local write "Module Admin"(w3) -> ()
  n179 = case "External Launch?" shown="True" w1 {
    tunnel: w13 -> [_ w437]
    frame False {
    }
    frame True {
      n180 = case shown="No Error" w437 {
        frame No Error {
          n181 = invoke class="VI" method="FP.Close"() -> ()  [unwired: 3 in, 3 out]
        }
        frame Error {
          n182 = invoke class="VI" method="FP.Open"("Activate"=TRUE ("Activate?")) -> ()  [unwired: 4 in, 5 out]
        }
      }
    }
  }
